vi "E816_Piezo_ctrl.vi"(2 "error in":errorcluster, 3 "Position values":dbl[](array[numeric])=[0.01]) -> (0 "error out":errorcluster, 1 "Position":dbl[](array[numeric]) format="%.6f")   [LabVIEW 2009]
doc: "This VI demonstrates how to initialize an E-816 system, how to move an axis and how to query for the position value of this axis.\n\nIn this example the E-816 is connected through COM port 1 with baudrate 57600. The VI runs E816_Configuration_Setup.vi with these specified settings, moves the first axis relative to its current position, waits for the movement to finish and reads the position of the axis and the error status of the controller. The diagram shows how to combine the driver VIs for these tasks. \n\nFor an example of how to command multiple axes through an USB connection see E816_Sample_ Application_1a.vi\n\nWarning: Before running this VI, modify the interface settings on the block diagram to reflect your configuration. The predefined settings provided with the VI probably do not match your system."
panel:
  in  "stop":bool
  out "Running":bool caption="Configuration_Setup.vi is running"
  out "First conn. axis":string[](array[string])
  out "Identification":string
  # "This VI demonstrates how to initialize an E-816 system, how to move an axis and how to query for the position value of this axis. \nThe VI runs E816_Configuration_Setup.vi with specified settings, moves the first axis relative to its current position and reads the\nposition of this axis. The diagram shows how to combine the driver VIs for these tasks. \n\nWarning: Before running this VI, modify the interface settings on the block diagram to reflect your configuration. The predefined \n                 settings provided with the VI probably do not match your system."
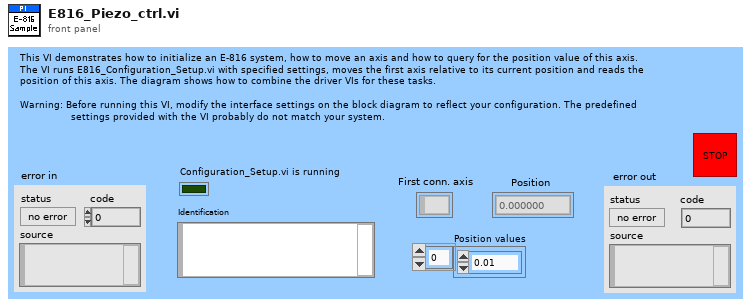
[diagram p1: front panel]
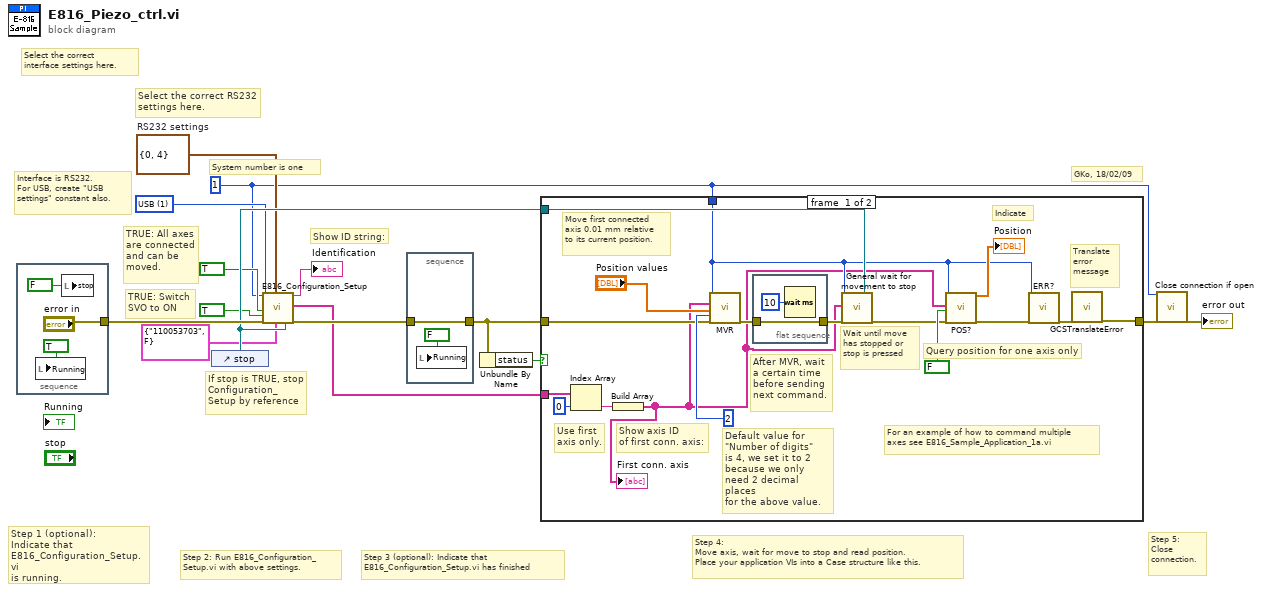
[diagram p0: block diagram]
diagram:
  w5 = u16 1 items=["RS232", "USB"] ("Interface")
  w8 = cluster{"Portnumber":i32, "Baudrate":u16} {"Portnumber"=0, "Baudrate"=4}  # RS232 settings
  w2 = 1 ("System no.")
  # "Select the correct\ninterface settings here."
  # "Step 5: \nClose\nconnection."
  # "Interface is RS232.\nFor USB, create \"USB\nsettings\" constant also."
  # "TRUE: All axes\nare connected\nand can be\nmoved."
  # "TRUE: Switch\nSVO to ON"
  # "If stop is TRUE, stop\nConfiguration_\nSetup by reference"
  # "Step 4: \nMove axis, wait for move to stop and read position.\nPlace your application VIs into a Case structure like this."
  # "Select the correct RS232\nsettings here."
  # "GKo, 18/02/09"
  # "Step 3 (optional): Indicate that \nE816_Configuration_Setup.vi has finished"
  # "Step 2: Run E816_Configuration_\nSetup.vi with above settings."
  # "Step 1 (optional): \nIndicate that \nE816_Configuration_Setup.vi\nis running."
  # "Show ID string:"
  # "System number is one"
  n1 = stacked-sequence {
    tunnel: ["error in"] -> w13
    frame #0 {
      n2 = local write "Running"(TRUE ("Running")) -> ()
      n3 = local write "stop"(FALSE ("stop")) -> ()
    }
  }
  n4 = control-ref of="stop"() -> (w10:refnum<vi>)
  n5 = call "E816_Configuration_Setup.vi"("System no."=w2, "Interface"=w5, "All axes?"=TRUE, "Change servo \nstatus to ON?"=TRUE ("Use dialog to define\nconnected stages?"), "error in"=w13, "RS232 settings"=w8, "USB settings"=cluster{"S/N":string, "USB Search?":bool} {"S/N"="110053703", "USB Search?"=FALSE}, "Stop refnum"=w10) -> ("Identification"=→"Identification":string, "Conn. Axes"=w9:string[], "error out"=w14:errorcluster)  [unwired: 3 in, 6 out]
  n6 = stacked-sequence {
    tunnel: w14 -> [w20]
    tunnel: [w20] -> w12
    frame #0 {
      n7 = local write "Running"(FALSE ("Running")) -> ()
    }
  }
  n8 = Unbundle By Name(w12) -> ("status"=w11:bool)
  n9 = case shown="False" w11 {
    tunnel: [w32 w40] -> w4
    tunnel: w9 -> [w24 _]
    tunnel: w2 -> [w28 _]
    tunnel: w12 -> [w33 w40]
    tunnel: w10 -> [w31 _]
    frame #0 {
      # "Show axis ID\nof first conn. axis:"
      # "For an example of how to command multiple\naxes see E816_Sample_Application_1a.vi"
      # "Use first\naxis only."
      # "After MVR, wait\na certain time\nbefore sending\nnext command."
      # "Translate\nerror \nmessage"
      # "Wait until move\nhas stopped or\nstop is pressed"
      # "Indicate"
      # "Default value for\n\"Number of digits\"\nis 4, we set it to 2\nbecause we only\nneed 2 decimal places\nfor the above value."
      # "Move first connected\naxis 0.01 mm relative\nto its current position."
      # "Query position for one axis only"
      n10 = Index Array(array=w24, index=0) -> (element=w22:string)
      n11 = Build Array(w22) -> (w21:string[])
      "First conn. axis" <- w21
      n12 = call "MVR.vi"("System no."=w28, "Axes to move"=w21, "Position values"="Position values", "No.of digits"=i16 2, "error in"=w33) -> ("error out"=w26:errorcluster)  [unwired: 14 out]
      n13 = flat-sequence {
        tunnel: w26 -> [w39]
        tunnel: [w39] -> w25
        frame #0 {
          n14 = Wait (ms)(milliseconds to wait=u32 10) -> ()  [unwired: 1 out]
        }
      }
      n15 = call "General wait for movement to stop.vi"("System no."=w28, "Axes to wait for"=w21, "error in"=w25, "Stop refnum"=w31) -> ("error out"=w27:errorcluster)  [unwired: 4 in, 11 out]
      n16 = call "POS?.vi"("System no."=w28, "Axes to query"=w21, "All axes?"=FALSE, "error in"=w27) -> ("Position"=→"Position":dbl[], "error out"=w30:errorcluster)  [unwired: 1 in, 13 out]
      n17 = call "ERR?.vi"("System no."=w28, "error in"=w30) -> ("error out"=w29:errorcluster)  [unwired: 17 out]
      n18 = call "GCSTranslateError.vi"("error in"=w29) -> ("error out"=w32:errorcluster)  [unwired: 18 out]
    }
    frame #1 {
      # "Error during initialization"
    }
  }
  n19 = call "Close connection if open.vi"("System no."=w2, "error in"=w4) -> ("error out"=→"error out":errorcluster)  [unwired: 1 in, 16 out]
